vi "Init Message.vi"(5 "TestManagerMsg":refnum<class "TestManagerMsg.lvclass">, 7 "overwrite?":bool=TRUE, 9 "key":string, 10 "self-id":string, 11 "owner-id":string) -> (3 "Message":refnum<class "TestManagerMsg.lvclass">)   [LabVIEW 2020, in "Caraya.lvlib" / "TestManagerMsg.lvclass"]
uses:
  TestManagerMsg.lvclass
  TestManagerMsg.lvclass/TestManagerMsg.ctl
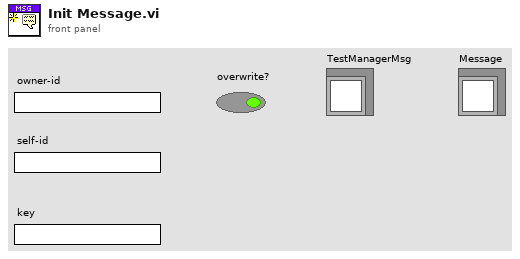
[diagram p1: front panel]
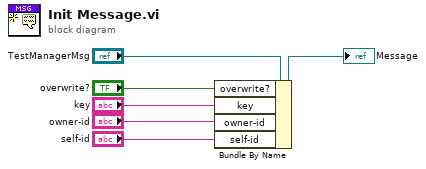
[diagram p0: block diagram]
diagram:
  n1 = Bundle By Name(cluster="TestManagerMsg", "overwrite?"="overwrite?", "key"="key", "owner-id"="owner-id", "self-id"="self-id") -> (→"Message":refnum<class "TestManagerMsg.lvclass">)
